vi "Initialize.vi"(8 "Error In":errorcluster) -> (0 "Error Out":errorcluster)   [LabVIEW 2019, in "Andor.lvlib"]
uses:
  Andor.lvlib
  Queues/Queues.lvlib
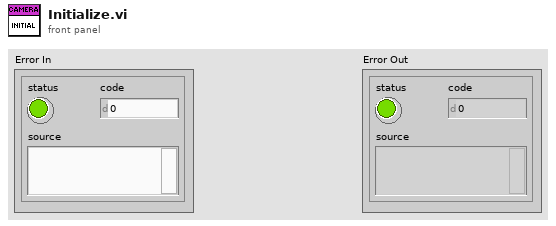
[diagram p1: front panel]
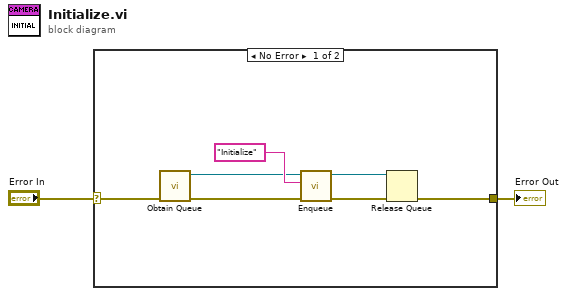
[diagram p0: block diagram]
diagram:
  n1 = case shown="No Error" "Error In" {
    selector: "Error In" -> [w8 w10]
    tunnel: [w4 w10] -> w2
    frame No Error {
      n2 = call "Obtain Queue.vi"("Error In"=w8) -> ("Error Out"=w7:errorcluster, "Queue out"=w6:refnum<queue>)  [unwired: 9 in]
      n3 = call "Enqueue.vi"("Error In"=w7, "State"="Initialize", "Queue in"=w6) -> ("Error Out"=w5:errorcluster, "Queue out"=w3:refnum<queue>)  [unwired: 7 in]
      n4 = Release Queue(queue=w3, error in (no error)=w5) -> (error out=w4:errorcluster)  [unwired: 1 in, 2 out]
    }
    frame Error {
    }
  }
  "Error Out" <- w2
